vi "Fix Offset.vi"(1 "Input Angle":dbl format="%#_13g") -> (0 "Output Angle":dbl)   [LabVIEW 2018]
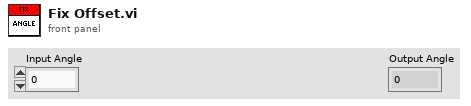
[diagram p1: front panel]
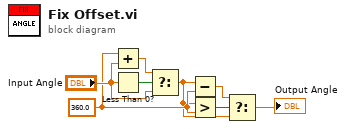
[diagram p0: block diagram]
diagram:
  w5 = 360.0
  n1 = Add(x=w5, y="Input Angle") -> (x+y=w6:dbl)
  n2 = Less Than 0?(x="Input Angle") -> (x < 0?=w8:bool)
  n3 = Select(t=w6, s=w8, f="Input Angle") -> (s? t:f=w2:dbl)
  n4 = Subtract(x=w2, y=w5) -> (x-y=w3:dbl)
  n5 = Greater?(x=w2, y=w5) -> (0:w4:bool)
  n6 = Select(t=w3, s=w4, f=w2) -> (s? t:f=→"Output Angle":dbl)
